vi "SubCalculate_TakeArrayColumnAverage.vi"(11 "2D-Array in":dbl[][](array[numeric])) -> (3 "Array Average of Column":dbl[](array[numeric]))   [LabVIEW 2015]
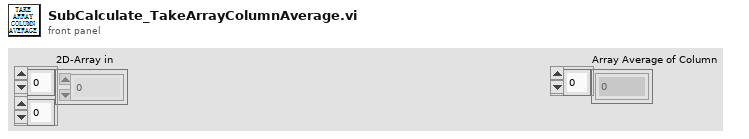
[diagram p1: front panel]
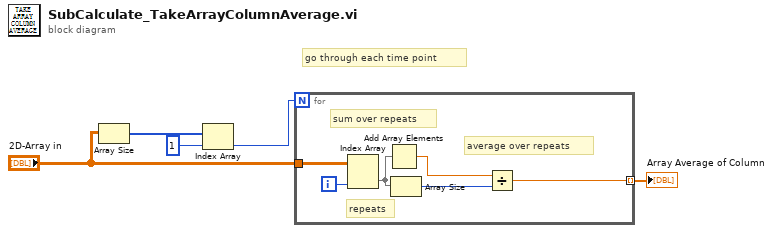
[diagram p0: block diagram]
diagram:
  # "go through each time point"
  n1 = Array Size(array="2D-Array in") -> (size(s)=w3:i32[])
  n2 = Index Array(array=w3, index=1) -> (element=w1:i32)
  n3 = for {
    N: w1 -> [_]
    tunnel: "2D-Array in" -> [w9]
    tunnel: [w7] -> w5 mode=indexing
    i -> [w6]
    # "average over repeats"
    # "repeats"
    # "sum over repeats"
    n4 = Index Array(array=w9, index (col)=w6) -> (element=w8:dbl[])  [unwired: 1 in]
    n5 = Add Array Elements(numeric array=w8) -> (sum=w11:dbl)
    n6 = Array Size(array=w8) -> (size(s)=w10:i32)
    n7 = Divide(x=w11, y=w10) -> (x/y=w7:dbl)
  }
  "Array Average of Column" <- w5
